vi "Main.vi"() -> ()   [LabVIEW 2019]
uses:
  <vilib>/Platform/TimedLoop/XDataNode/timing_clust.ctl
  <vilib>/Platform/TimedLoop/XDataNode/nitl_modes.ctl
  <vilib>/Platform/TimedLoop/XDataNode/wakeup.ctl
  <vilib>/myRIO/Instrument Drivers/Onboard IO/PWM/typedefs/PWM Reference.ctl
  <vilib>/myRIO/Common/Instrument Driver Framework/Utilities/typedefs/myRIO Generic Hardware Reference.ctl
  <vilib>/myRIO/Common/Instrument Driver Framework/Utilities/typedefs/Hardware Version Enum.ctl
  <vilib>/myRIO/Common/Instrument Driver Framework/Utilities/typedefs/myRIO v1.0 Reference.ctl
  <vilib>/myRIO/Common/Instrument Driver Framework/Utilities/typedefs/Generic FPGA Reference.ctl
  <vilib>/myRIO/Common/Instrument Driver Framework/myRIO v1.0/PWM/typedefs/PWM Channels Enum.ctl
  <vilib>/myRIO/Instrument Drivers/Onboard IO/PWM/typedefs/PWM Configuration.ctl
  <vilib>/userDefined/High Color/nirio_resource_hc.ctl
  <vilib>/myRIO/Instrument Drivers/Onboard IO/DIO/typedefs/DIO Reference.ctl
  <vilib>/myRIO/Common/Instrument Driver Framework/myRIO v1.0/DIO/typedefs/DIO Channels List.ctl
  <vilib>/myRIO/Common/Instrument Driver Framework/myRIO v1.0/DIO/typedefs/DIO Channels Enum.ctl
  <vilib>/myRIO/Common/Instrument Driver Framework/Utilities/vis/Is FPGA Ref Available.vi
  <vilib>/myRIO/Common/Instrument Driver Framework/myRIO v1.0/PWM/vis/myRIO v1.1 Open PWM.vi
  <vilib>/myRIO/Instrument Drivers/Onboard IO/PWM/vis/Set Duty Cycle and Frequency.vi
  <vilib>/myRIO/Common/Instrument Driver Framework/myRIO v1.0/DIO/vis/myRIO v1.1 Open DIO.vi
  <extravilib>/ChannelInstances/Tag-bool/Write With Abort.vi
  <extravilib>/ChannelInstances/Tag-bool/Read With Abort.vi
  <vilib>/myRIO/Common/Instrument Driver Framework/Utilities/vis/Validate Channels.vi
  <vilib>/myRIO/Common/Instrument Driver Framework/myRIO v1.0/PWM/vis/myRIO v1.0 Reserve PWM.vi
  <vilib>/myRIO/Common/Instrument Driver Framework/myRIO v1.0/DIO/vis/myRIO v1.0 Reserve DIO.vi
  <vilib>/myRIO/Common/Instrument Driver Framework/myRIO v1.0/I2C/vis/myRIO v1.0 Close I2C.vi
  <vilib>/myRIO/Common/Instrument Driver Framework/myRIO v1.0/UART/vis/myRIO v1.0 Close UART.vi
  <vilib>/myRIO/Common/Instrument Driver Framework/myRIO v1.0/PWM/vis/myRIO v1.0 Build MUX Configuration PWM.vi
  <vilib>/myRIO/Common/Instrument Driver Framework/myRIO v1.0/Resource Manager/vis/myRIO v1.0 Reserve Channel List.vi
  <vilib>/myRIO/Common/Instrument Driver Framework/myRIO v1.0/DIO/vis/myRIO v1.0 Build MUX Configuration DIO.vi
  <vilib>/myRIO/Common/Instrument Driver Framework/myRIO v1.0/I2C/vis/myRIO v1.0 Unreserve I2C.vi
  <vilib>/myRIO/Common/Instrument Driver Framework/myRIO v1.0/Resource Manager/vis/myRIO v1.0 Create Configuration List.vi
  <vilib>/myRIO/Common/Instrument Driver Framework/myRIO v1.0/Resource Manager/vis/myRIO v1.0 Reserve Channel.vi
  <vilib>/myRIO/Common/Instrument Driver Framework/myRIO v1.0/Resource Manager/vis/myRIO v1.0 Unreserve Channel.vi
  <vilib>/myRIO/Common/Instrument Driver Framework/myRIO v1.0/I2C/vis/myRIO v1.0 Build MUX Configuration I2C.vi
  <vilib>/myRIO/Common/Instrument Driver Framework/myRIO v1.0/Resource Manager/vis/myRIO v1.0 Unreserve Channel List.vi
  <vilib>/myRIO/Common/Instrument Driver Framework/myRIO v1.0/Resource Manager/vis/myRIO v1.0 Build Mutex Name.vi
  <extravilib>/ChannelInstances/Tag-bool/Instantiate.vi
  <extravilib>/ChannelInstances/Tag-bool/EndpointRead.vi
  <vilib>/Utility/VariantDataType/GetNumericInfo.vi
  <vilib>/Utility/error.llb/Error Cluster From Error Code.vi
  <vilib>/myRIO/Common/Instrument Driver Framework/myRIO v1.0/myRIO v1.1 Open.vi
  <vilib>/myRIO/Common/Instrument Driver Framework/Utilities/vis/IO Manager.vi
  <vilib>/myRIO/Common/Instrument Driver Framework/Utilities/vis/Configuration Manager.vi
  <vilib>/myRIO/Common/Instrument Driver Framework/myRIO v1.0/Resource Manager/vis/myRIO v1.0 Configure IO.vi
  <vilib>/myRIO/Common/Instrument Driver Framework/myRIO v1.0/myRIO v1.0 Close.vi
  <vilib>/myRIO/Common/Instrument Driver Framework/myRIO v1.0/PWM/vis/myRIO v1.0 Write PWM.vi
  <vilib>/myRIO/Common/Instrument Driver Framework/myRIO v1.0/DIO/vis/myRIO v1.0 Write DIO.vi
  <vilib>/myRIO/Common/Instrument Driver Framework/myRIO v1.0/I2C/vis/myRIO v1.0 Shutdown I2C.vi
  <vilib>/rvi/errors/niLvFpgaAdjustHostInterfaceError.vi
  <vilib>/FPGAPlugInAG/Dynamic/niLvFpga_Abort_Dynamic.vi
  <vilib>/myRIO/Common/Instrument Driver Framework/Utilities/vis/FPGA Ref Manager.vi
  <vilib>/myRIO/Common/Instrument Driver Framework/myRIO v1.0/myRIO v1.0 Reset FPGA.vi
  <vilib>/myRIO/Common/Instrument Driver Framework/myRIO v1.0/IRQ/vis/myRIO v1.0 IRQ Info FGV.vi
  <vilib>/myRIO/Common/Instrument Driver Framework/myRIO v1.0/IRQ/vis/myRIO v1.0 Timer IRQ Info FGV.vi
  <vilib>/myRIO/Common/Instrument Driver Framework/myRIO v1.0/IRQ/vis/myRIO v1.0 ISR Agent.vi
  <vilib>/myRIO/Instrument Drivers/Utilities/vis/Reset Index.vi
  <vilib>/myRIO/Common/Instrument Driver Framework/myRIO v1.0/Resource Manager/vis/myRIO v1.0 Block Write Resource Manager.vi
  <vilib>/FPGAPlugInAG/Dynamic/niLvFpga_Close_Dynamic.vi
  <extravilib>/ChannelInstances/Tag-bool/Endpoint.vi
  <vilib>/platform/TimedLoop/XDataNode/XDataNode.xnode
  <vilib>/myRIO/Express VI/Onboard IO/PWM/PWM Express VI.xnode
  <vilib>/myRIO/Instrument Drivers/Onboard IO/PWM/vis/myRIO PWM Open.xnode
  <vilib>/myRIO/Express VI/Onboard IO/DO/DO Express VI.xnode
  <vilib>/myRIO/Instrument Drivers/Onboard IO/DIO/vis/myRIO DIO Open.xnode
  <vilib>/rvi/interface/nirviReadWriteControl/nirviReadWriteControl.xnode
  <vilib>/rvi/interface/nirviMethod/nirviMethod.xnode
  <vilib>/rvi/interface/nirviCloseFPGA/nirviCloseFPGA.xnode
  <vilib>/rvi/interface/Simulation/niFpgaSimulationCallBeginRW.vi
  <vilib>/Platform/TimedLoop/XDataNode/XDNodeRunTimeDep.lvlib
  <vilib>/myRIO/Instrument Drivers/Utilities/Utilities.lvlib
  NiFpgaLv.dll
  <extravilib>/ChannelInstances/Tag-bool.lvlib
  <vilib>/myRIO/Instrument Drivers/Onboard IO/PWM/PWM.lvlib
  <vilib>/myRIO/Instrument Drivers/Onboard IO/DIO/DIO.lvlib
  <vilib>/myRIO/Instrument Drivers/Onboard IO/I2C/I2C.lvlib
panel:
  out "Encoder Position (Degrees) 2":dbl
  out "Duty Cycle PWM":dbl(graph)
  in  "Inner PID T/F":bool
  in  "D_i":dbl
  in  "I_i":dbl
  in  "P_i":dbl
  in  "Log file path":path
  out "Duty Cycle":dbl
  in  "Angle limit (degrees)":i32
  in  "D_o":dbl
  in  "I_o":dbl
  in  "P_o":dbl
  in  "Speed (km/h)":dbl
  out "Combined loop duration time (us)":i64
  in  "Loop durations":T1(tab)
  out "IMU Data gathering duration(us)":i64(graph)
  out "Encoder data gathering duration(us)":i64(graph)
  out "Steering Motor duration(us)":i64(graph)
  out "E-Stop loop duration (us)":i64(graph)
  in  "GO":bool
  in  "E-stop":bool
  out "Indicator":bool
  in  "Encoder Position Reset":bool
  out "Encoder Velocity (deg/s)":dbl
  out "Encoder Acceleration (deg/s^2)":dbl
  out "Encoder Position (Degrees)":dbl
  out "IMU Gyro Chart":cluster{dbl, dbl, dbl}(graph)
  out "IMU Acc Chart":cluster{dbl, dbl, dbl}(graph)
  # "Steering Motor"
  # "Forward Motor"
  # "Outer"
  # "(2)"
  # "Inner"
  # "Start Motors"
  # "(3)"
  # "(1)"
  # "(4)"
  # "(6)"
  # "(7)"
  # "(5)"
  # "(8)"
  # "(8)"
  # "(8)"
  # "(8)"
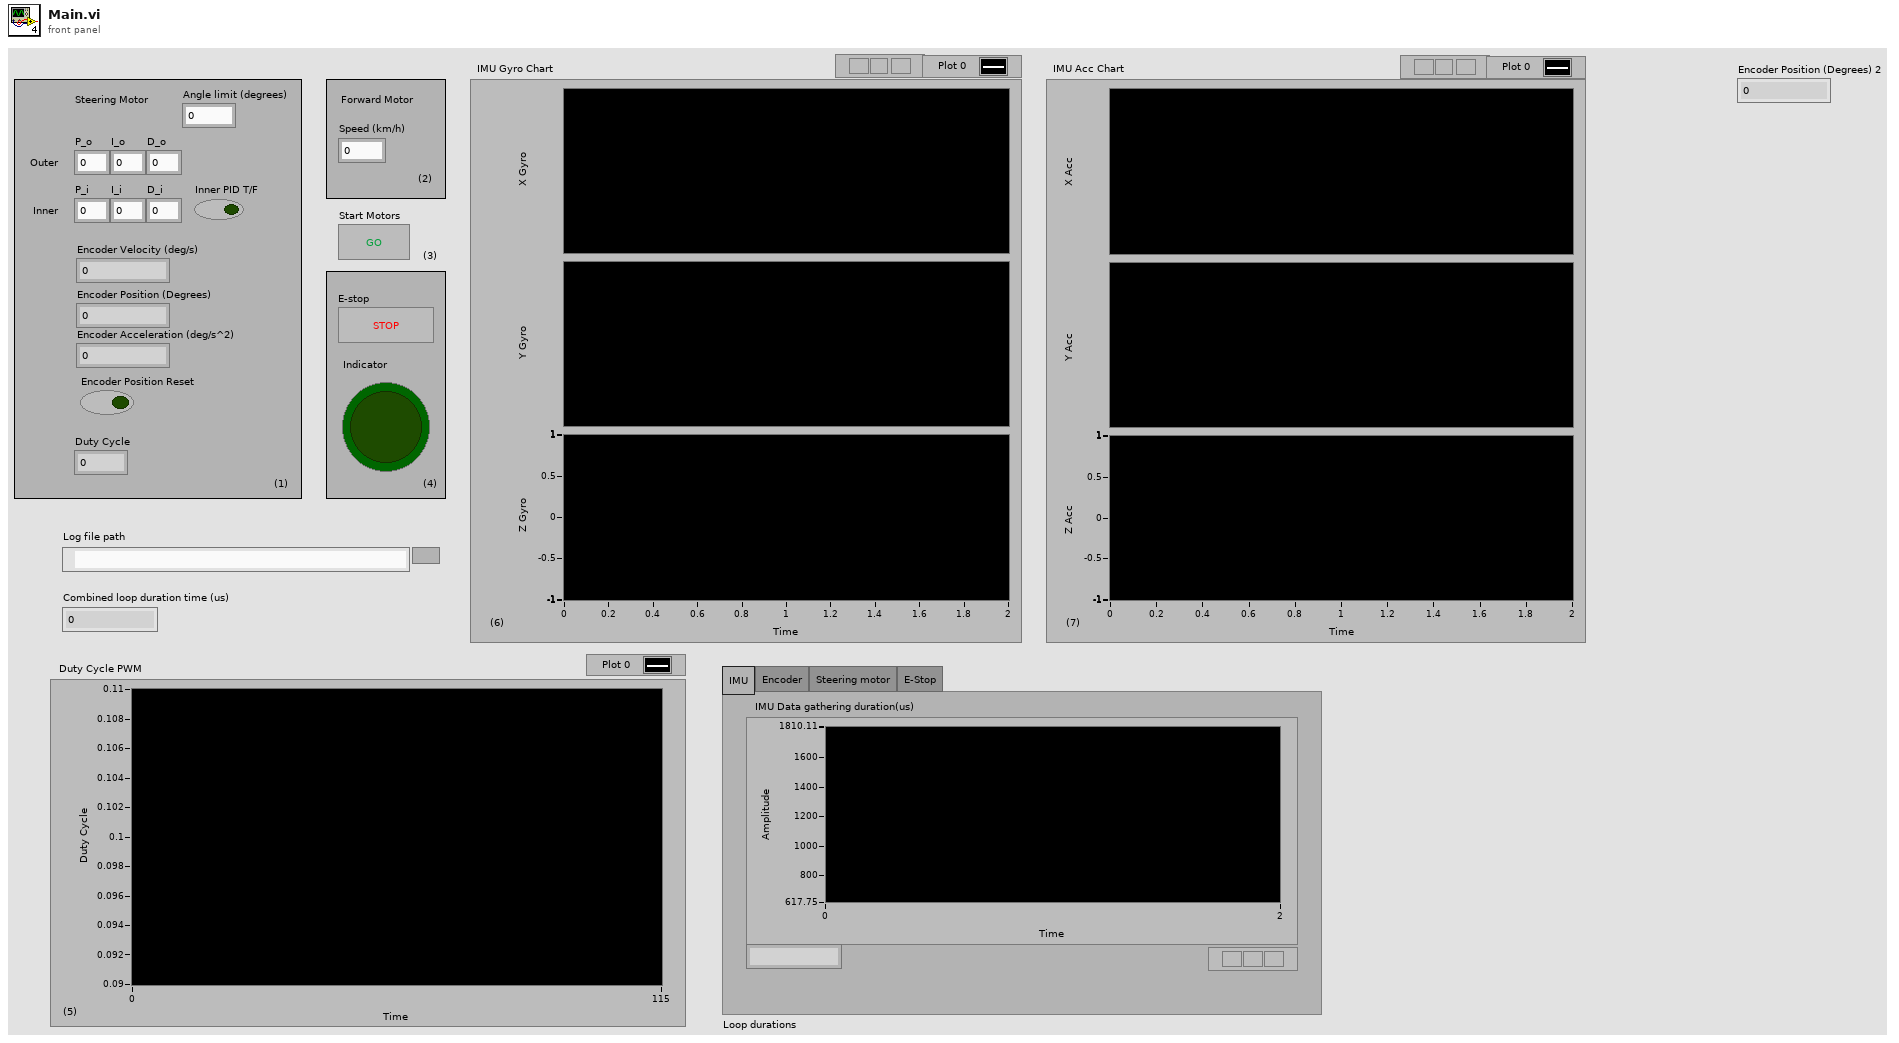
[diagram p1: front panel]
types:
  T1 = enum32{"IMU", "Encoder", "Steering motor", "E-Stop"}
  T2 = enum16{"open", "open or create", "create or replace", "create", "open (read-only)"}
  T3 = typedef "XDNodeRunTimeDep.lvlib/timing_clust.ctl" = cluster{"Expected End [f-1]":u64, "Actual End [f-1]":u64, "Finished Late? [f-1]":bool, "Expected End [i-1]":u64, "Actual End [i-1]":u64, "Finished Late? [i-1]":bool, "Expected Start [i]":u64, "Actual Start [i]":u64, "Expected Start [f]":u64, "Actual Start [f]":u64, "Source Name":string, "Structure Name":string, "Period":i64, "Deadline":i64, "Offset":i64, "Start":i64, "Priority":i32, "Timeout":i32, "Mode":T4, "Wakeup Reason":T5, "Error":errorcluster, "Source Type":string, "Secondary Source Type":string, "Global End Time":u64, "Global Start Time":u64, "Frame Duration":u64, "Iteration Duration":u64, "Assigned CPU":i32, "I/O Scan Engine Mode":u32}
  T4 = typedef "XDNodeRunTimeDep.lvlib/nitl_modes.ctl" = enum32{"No Change", "Process missed periods, maintain original phase", "Discard missed periods, maintain original phase", "Process missed periods, ignore original phase", "Discard missed periods, ignore original phase"}
  T5 = typedef "XDNodeRunTimeDep.lvlib/wakeup.ctl" = enum32{"Normal", "Aborted", "Asynchronous wakeup", "Timing source error", "Timed loop error", "Timeout"}
  T6 = typedef "I2C.lvlib/I2C Reference.ctl" = cluster{"myRIO Reference":T7, "I2C Channels Enum":T11, "I2C Configuration":T12}
  T7 = typedef "myRIO Generic Hardware Reference.ctl" = cluster{"myRIO Model":T8, "myRIO Hardware Reference":T9}
  T8 = typedef "Hardware Version Enum.ctl" = enum16{"Unknown", "myRIO-1900", "myRIO-1950", "roboRIO", "NI ELVIS RIO CM", "ELVIS III"}
  T9 = typedef "myRIO v1.0 Reference.ctl" = cluster{"Generic FPGA Reference":T10, "Allow multiple opens":bool}
  T10 = typedef "Generic FPGA Reference.ctl" = refnum<k20>
  T11 = typedef "I2C Channels Enum.ctl" = enum16{"Not Connected", "A/I2C", "B/I2C", "I2C/I2C"}
  T12 = typedef "I2C.lvlib/I2C Configuration.ctl" = cluster{"I2C Transfer Rate":T13}
  T13 = typedef "I2C.lvlib/I2C Transfer Rate.ctl" = enum16{"Standard mode (100 kbps)", "Fast mode (400 kbps)"}
  T14 = typedef "Tag-bool.lvlib/))Channel.ctl" = refnum<queue>
  T15 = typedef "PWM.lvlib/PWM Reference.ctl" = cluster{"myRIO Reference":T7, "PWM Channels Enum":T16, "PWM Configuration":T17}
  T16 = typedef "PWM Channels Enum.ctl" = enum16{"Not Connected", "C/PWM0", "C/PWM1", "A/PWM0", "A/PWM1", "A/PWM2", "A/PWM3", "A/PWM4", "A/PWM5", "A/PWM6", "A/PWM7", "A/PWM8", "A/PWM9", "A/PWM10", "A/PWM11", "A/PWM12", "A/PWM13", "A/PWM14", "A/PWM15", "A/PWM16", "A/PWM17", "A/PWM18", "A/PWM19", "B/PWM0", "B/PWM1", "B/PWM2", "B/PWM3", "B/PWM4", "B/PWM5", "B/PWM6", "B/PWM7", "B/PWM8", "B/PWM9", "B/PWM10", "B/PWM11", "B/PWM12", "B/PWM13", "B/PWM14", "B/PWM15", "B/PWM16", "B/PWM17", "B/PWM18", "B/PWM19", "PWM/PWM0", "PWM/PWM1", "PWM/PWM2", "PWM/PWM3", "PWM/PWM4", "PWM/PWM5", "PWM/PWM6", "PWM/PWM7", "PWM/PWM8", "PWM/PWM9"}
  T17 = typedef "PWM.lvlib/PWM Configuration.ctl" = cluster{"Frequency":dbl, "Duty Cycle":dbl}
  T18 = typedef "nirio_resource_hc.ctl" = tag
  T19 = typedef "DIO.lvlib/DIO Reference.ctl" = cluster{"myRIO Reference":T7, "DIO Channels List":T20}
  T20 = typedef "DIO Channels List.ctl" = T21[]
  T21 = typedef "DIO Channels Enum.ctl" = enum16{"Not Connected", "C/DIO0", "C/DIO1", "C/DIO2", "C/DIO3", "C/DIO4", "C/DIO5", "C/DIO6", "C/DIO7", "A/DIO0", "A/DIO1", "A/DIO2", "A/DIO3", "A/DIO4", "A/DIO5", "A/DIO6", "A/DIO7", "A/DIO8", "A/DIO9", "A/DIO10", "A/DIO11", "A/DIO12", "A/DIO13", "A/DIO14", "A/DIO15", "A/DIO16", "A/DIO17", "A/DIO18", "A/DIO19", "B/DIO0", "B/DIO1", "B/DIO2", "B/DIO3", "B/DIO4", "B/DIO5", "B/DIO6", "B/DIO7", "B/DIO8", "B/DIO9", "B/DIO10", "B/DIO11", "B/DIO12", "B/DIO13", "B/DIO14", "B/DIO15", "B/DIO16", "B/DIO17", "B/DIO18", "B/DIO19", "LED0", "LED1", "LED2", "LED3", "Button0", "DIO/DIO0", "DIO/DIO1", "DIO/DIO2", "DIO/DIO3", "DIO/DIO4", "DIO/DIO5", "DIO/DIO6", "DIO/DIO7", "DIO/DIO8", "DIO/DIO9", "SPI/CS0", "SPI/CS1", "SPI/CS2", "SPI/CS3", "LED RADIO (Green)", "LED RADIO (Red)", "LED COMM (Green)", "LED COMM (Red)", "LED MODE (Green)", "LED MODE (Red)"}
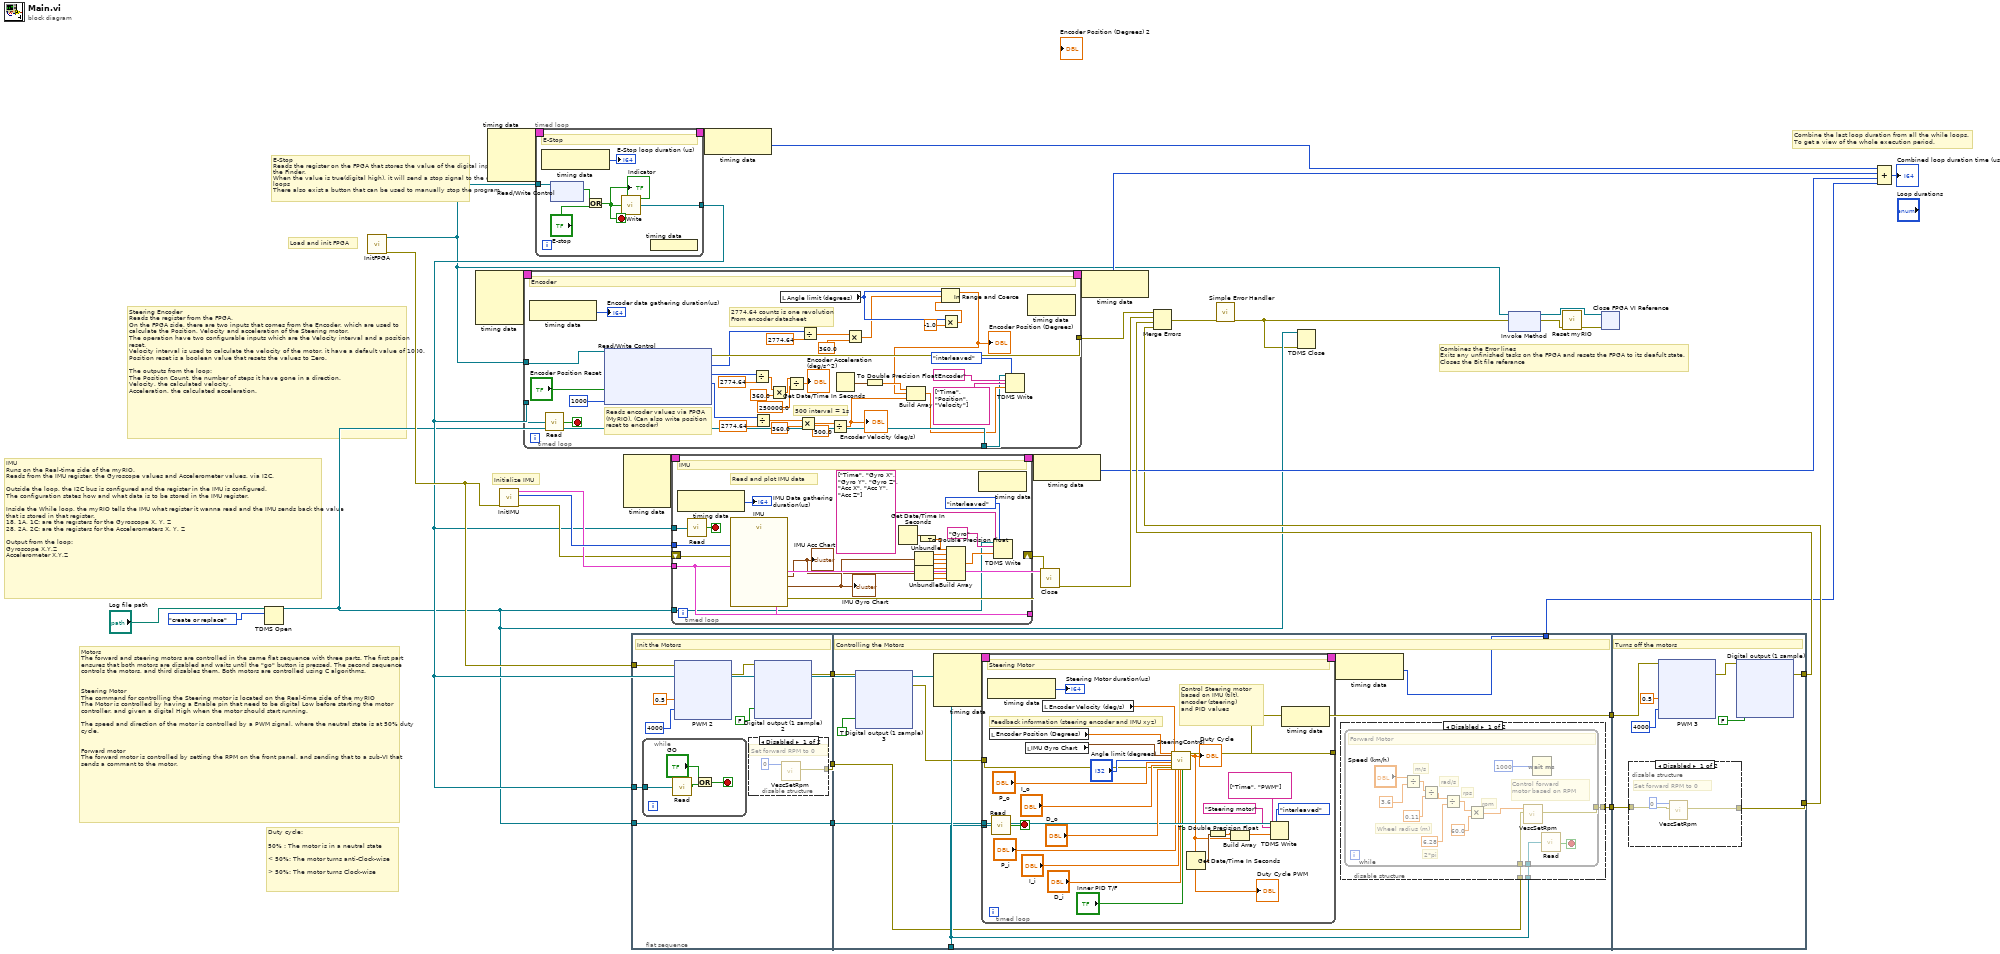
[diagram p0: block diagram]
diagram:
  # "Duty cycle:\n\n50% : The motor is in a neutral state\n\n< 50%: The motor turns anti-Clock-wise\n\n> 50%: The motor turns Clock-wise"
  # "Initialize IMU"
  # "Load and init FPGA"
  # "Combines the Error lines\nExits any unfinished tasks on the FPGA and resets the FPGA to its deafult state.\nCloses the Bit file referance"
  # "Combine the last loop duration from all the while loops.\nTo get a view of the whole execution period."
  # "Motors\nThe forward and steering motors are controlled in the same flat sequence with three parts. The first part ensures that both motors are disabled and waits until the \"go\" button is pressed. The second sequence controls the motors, and third disables them. Both motors are controlled using C algorithms.\n\n\nSteering Motor\nThe command for controlling the Steering motor is located on the Real-time side of the myRIO\nThe Motor is controlled by having a Enable pin that need to be digital Low before starting the motor controller, and given a digital High when the motor should start running.\n\nThe speed and direction of the motor is controlled by a PWM signal, where the neutral state is at 50% duty cycle.\n\n\nForward motor\nThe forward motor is controlled by setting the RPM on the front panel, and sending that to a sub-VI that sends a commant to the motor."
  # "IMU\nRuns on the Real-time side of the myRIO.\nReads from the IMU register, the Gyroscope values and Accelerometer values, via I2C.\n\nOutside the loop, the I2C bus is configured and the register in the IMU is configured.\nThe configuration states how and what data is to be stored in the IMU register.\n\nInside the While loop, the myRIO tells the IMU what register it wanna read and the IMU sends back the value that is stored in that register.\n18, 1A, 1C: are the registers for the Gyroscope X, Y, Z\n28, 2A, 2C: are the registers for the Accelerometers X, Y, Z\n\nOutput from the loop:\nGyroscope X,Y,Z\nAccelerometer X,Y,Z"
  # "Steering Encoder\nReads the register from the FPGA. \nOn the FPGA side, there are two inputs that comes from the Encoder, which are used to calculate the Position, Velocity and acceleration of the Steering motor.\nThe operation have two configurable inputs which are the Velocity interval and a position reset.\nVelocity interval is used to calculate the velocity of the motor, it have a default value of 1000.\nPosition reset is a boolean value that resets the values to Zero.\n\nThe outputs from the loop:\nThe Position Count, the number of steps it have gone in a direction. \nVelocity, the calculated velocity.\nAcceleration, the calculated acceleration."
  # "E-Stop\nReads the register on the FPGA that stores the value of the digital input from the Finder.\nWhen the value is true(digital high), it will send a stop signal to the other while loops\nThere also exist a button that can be used to manually stop the program."
  n1 = TDMS Open(10:T2."create or replace" ("operation (0:open)"), 11:"Log file path") -> (3:w5:refnum<k34>)  [unwired: 5 in, 1 out]
  n2 = call "InitFPGA.vi"() -> ("error out"=w20:errorcluster, "Refnum out"=w1:refnum<k20>)  [unwired: 10 in]
  n3 = node-c288() -> (w33:T3)  [unwired: 4 in]
  n4 = node-c288() -> (w27:T3)  [unwired: 4 in]
  n5 = call "InitIMU.vi"("error in (no error)"=w20) -> ("error out"=w15:errorcluster, "Acc/Gyro  address"=w22:u8, "I2C Ref Out"=w21:T6)  [unwired: 8 in]
  n6 = timed-loop {
    timing: w27 -> [_]
    timing-out: [_] -> w26
    tunnel: w1 -> [w42]
    tunnel: [w41] -> w13
    stop <- w37 stop-if-true
    # "E-Stop"
    n7 = node-c288() -> (→"E-Stop loop duration (us)":i64)  [unwired: 1 in]
    n8 = xnode "Read/Write Control"("FPGA VI Reference In"=w42) -> ("E-Stop"=w40:bool)  [unwired: 1 in, 2 out]
    n9 = Or(x=w40, y="E-stop") -> (x .or. y?=w37:bool)
    "Indicator" <- w37
    n10 = call <vilib>:"Write.vi"("element"=w37) -> ("channel"=w41:T14)  [unwired: 1 out]
    n11 = node-c288() -> ()  [unwired: 1 out]
  }
  n12 = timed-loop {
    timing: w33 -> [_]
    timing-out: [_] -> w32
    tunnel: w1 -> [w82]
    tunnel: [w81] -> w31
    tunnel: w13 -> [w77]
    tunnel: w5 -> [w72]
    stop <- w76 stop-if-true
    # "500 interval = 1s"
    # "2774,64 counts is one revolution\nFrom encoder datasheet"
    # "Reads encoder values via FPGA\n(MyRIO). (Can also write position\nreset to encoder)"
    # "Encoder"
    n13 = node-c288() -> (→"Encoder data gathering duration(us)":i64)  [unwired: 1 in]
    n14 = call <extravilib>:"Read.vi"("channel"=w77) -> ("element"=w76:bool)  [unwired: 1 in, 1 out]
    n15 = xnode "Read/Write Control"("FPGA VI Reference In"=w82, "Position Reset"="Encoder Position Reset", "Velocity Interval (uSec)"=u32 1000) -> ("error out"=w81:errorcluster, "Position (Counts)"=w68:i32, "Acceleration (Counts/Interval)"=w56:i32, "Velocity (Counts/Interval)"=w61:i32)  [unwired: 1 in, 1 out]
    n16 = Divide(x=w56, y=2774.64) -> (x/y=w54:dbl)
    n17 = Divide(x=w61, y=2774.64) -> (x/y=w62:dbl)
    n18 = Multiply(x=w54, y=360.0) -> (x*y=w53:dbl)
    n19 = local read "Angle limit (degrees)"() -> (w49:i32)
    n20 = Divide(x=w53, y=250000.0) -> (x/y=→"Encoder Acceleration (deg/s^2)":dbl)
    n21 = Multiply(x=w62, y=360.0) -> (x*y=w60:dbl)
    n22 = Divide(x=w68, y=2774.64) -> (x/y=w65:dbl)
    n23 = Divide(x=w60, y=500.0) -> (x/y=w58:dbl)
    "Encoder Velocity (deg/s)" <- w58
    n24 = Get Date/Time In Seconds() -> (seconds since 1Jan1904=w70:timestamp)
    n25 = Multiply(x=w65, y=360.0) -> (x*y=w47:dbl)
    n26 = To Double Precision Float(number=w70) -> (double precision float=w71:dbl)
    n27 = Multiply(x=w49, y=-1.0) -> (x*y=w50:dbl)
    n28 = In Range and Coerce(upper limit=w49, x=w47, lower limit=w50) -> (coerced(x)=w46:dbl)  [unwired: 1 out]
    "Encoder Position (Degrees)" <- w46
    n29 = Build Array(w71, w46, w58) -> (w73:dbl[])
    n30 = TDMS Write(0:w72, 1:enum16{"decimated", "interleaved"}."interleaved" ("data layout (0:decimated)"), 5:"Encoder" ("group name in (Untitled)"), 7:string[] ["Time", "Position", "Velocity"] ("channel name(s) in (Untitled)"), 9:w73) -> ()  [unwired: 1 in, 4 out]
    n31 = node-c288() -> ()  [unwired: 1 in, 1 out]
  }
  n32 = node-c288() -> (w29:T3)  [unwired: 4 in]
  n33 = flat-sequence {
    tunnel: [w93] -> w25
    tunnel: w20 -> [w91]
    tunnel: w13 -> [w89]
    tunnel: [w87] -> w12
    tunnel: w5 -> [w88]
    tunnel: [w88] -> w6
    tunnel: w25 -> [w181]
    tunnel: [w178] -> w3
    tunnel: w13 -> [w175]
    tunnel: w12 -> [w171]
    tunnel: [w174] -> w11
    tunnel: [w173] -> w9
    tunnel: w6 -> [w172]
    tunnel: [w270] -> w17
    tunnel: w11 -> [w266]
    tunnel: [w264] -> w10
    tunnel: w9 -> [w265]
    frame #0 {
      # "Init the Motors"
      n34 = while {
        tunnel: w89 -> [w97]
        stop <- w100 stop-if-true
        n35 = call <extravilib>:"Read.vi"("channel"=w97) -> ("element"=w98:bool)  [unwired: 1 in, 1 out]
        n36 = Or(x="GO", y=w98) -> (x .or. y?=w100:bool)
      }
      n37 = xnode "PWM 2"("Duty Cycle"=0.5, "Frequency [Hz]"=4000, "error in (no error)"=w91) -> ("error out"=w94:errorcluster)
      n38 = disable-structure shown="Disabled" {
        disable-tunnel: [w95 _] -> w87
        frame Disabled {
          # "Set forward RPM to 0"
          n39 = call "VescSetRpm.vi"("Speed (rpm)"=0) -> ("error out"=w95:errorcluster)  [unwired: 10 in]
        }
        frame Enabled {
        }
      }
      n40 = xnode "Digital output (1 sample) 2"("B/DIO4 (Pin 19)"=FALSE ("B/DIO1 (Pin 13)"), "error in (no error)"=w94) -> ("error out"=w93:errorcluster)
    }
    frame #1 {
      # "Controlling the Motors"
      n41 = xnode "Digital output (1 sample) 3"("B/DIO4 (Pin 19)"=TRUE ("B/DIO1 (Pin 13)"), "error in (no error)"=w181) -> ("error out"=w177:errorcluster)
      n42 = node-c288() -> (w180:T3)  [unwired: 4 in]
      n43 = timed-loop {
        tunnel: w177 -> [w199]
        timing: w180 -> [_]
        timing-out: [_] -> w179
        tunnel: w175 -> [w215]
        tunnel: [w213] -> w173
        tunnel: w172 -> [w212]
        stop <- w222 stop-if-true
        # "Feedback information (steering encoder and IMU xyz)"
        # "Control Steering motor\nbased on IMU (tilt), \nencoder (steering)\nand PID values"
        # "Steering Motor"
        n44 = node-c288() -> (→"Steering Motor duration(us)":i64)  [unwired: 1 in]
        n45 = local read "Encoder Position (Degrees)"() -> (w219:dbl)
        n46 = call <extravilib>:"Read.vi"("channel"=w215) -> ("element"=w222:bool)  [unwired: 1 in, 1 out]
        n47 = local read "IMU Gyro Chart"() -> (w220:cluster{dbl, dbl, dbl})
        n48 = local read "Encoder Velocity (deg/s)"() -> (w201:dbl)
        n49 = call "SteeringControl.vi"("Position (Degrees)"=w219, "Cluster"=w220, "Limit (degrees)"="Angle limit (degrees)", "P_o gain"="P_o", "I_o gain"="I_o", "error in (no error)"=w199, "D_o gain"="D_o", "Velocity (deg/s)"=w201, "P_i gain"="P_i", "I_i gain"="I_i", "D_i gain"="D_i", "Inner PID T/F"="Inner PID T/F") -> ("error out"=w213:errorcluster, "PWM Out"=w200:dbl)  [unwired: 14 in]
        "Duty Cycle" <- w200
        "Duty Cycle PWM" <- w200
        n50 = Get Date/Time In Seconds() -> (seconds since 1Jan1904=w208:timestamp)
        n51 = To Double Precision Float(number=w208) -> (double precision float=w209:dbl)
        n52 = Build Array(w209, w200) -> (w210:dbl[])
        n53 = TDMS Write(0:w212, 1:enum16{"decimated", "interleaved"}."interleaved" ("data layout (0:decimated)"), 5:"Steering motor" ("group name in (Untitled)"), 7:string[] ["Time", "PWM"] ("channel name(s) in (Untitled)"), 9:w210) -> ()  [unwired: 1 in, 4 out]
        n54 = node-c288() -> ()  [unwired: 1 in, 1 out]
      }
      n55 = node-c288(w179) -> (w178:i64)
      n56 = disable-structure shown="Disabled" {
        disable-tunnel: w175 -> [w184 _]
        disable-tunnel: [w183 _] -> w174
        disable-tunnel: w171 -> [w182 _]
        frame Disabled {
          n57 = while "Timed Loop" {
            tunnel: w184 -> [w197]
            tunnel: w182 -> [w186]
            tunnel: [w185] -> w183
            stop <- w198 stop-if-true
            # "2*pi"
            # "rpm"
            # "rps"
            # "rad/s"
            # "Wheel radius (m)"
            # "m/s"
            # "Control forward\nmotor based on RPM"
            # "Forward Motor"
            n58 = Divide(x="Speed (km/h)", y=3.6) -> (x/y=w193:dbl)
            n59 = Divide(x=w193, y=0.11) -> (x/y=w191:dbl)
            n60 = Divide(x=w191, y=6.28) -> (x/y=w190:dbl)
            n61 = Multiply(x=w190, y=60.0) -> (x*y=w188:dbl)
            n62 = call "VescSetRpm.vi"("error in (no error)"=w186, "Speed (rpm)"=w188) -> ("error out"=w185:errorcluster)  [unwired: 9 in]
            n63 = Wait (ms)(milliseconds to wait=1000) -> ()  [unwired: 1 out]
            n64 = call <extravilib>:"Read.vi"("channel"=w197) -> ("element"=w198:bool)  [unwired: 1 in, 1 out]
          }
        }
        frame Enabled {
        }
      }
    }
    frame #2 {
      # "Turns off the motors"
      n65 = disable-structure shown="Disabled" {
        disable-tunnel: w266 -> [w273 _]
        disable-tunnel: [w272 _] -> w264
        frame Disabled {
          # "Set forward RPM to 0"
          n66 = call "VescSetRpm.vi"("error in (no error)"=w273, "Speed (rpm)"=0) -> ("error out"=w272:errorcluster)  [unwired: 9 in]
        }
        frame Enabled {
        }
      }
      n67 = xnode "PWM 3"("Duty Cycle"=0.5, "Frequency [Hz]"=4000, "error in (no error)"=w265) -> ("error out"=w268:errorcluster)
      n68 = xnode "Digital output (1 sample)"("B/DIO4 (Pin 19)"=FALSE ("B/DIO1 (Pin 13)"), "error in (no error)"=w268) -> ("error out"=w270:errorcluster)
    }
  }
  n69 = timed-loop {
    timing: w29 -> [_]
    timing-out: [_] -> w28
    tunnel: w22 -> [w366]
    tunnel: w21 -> [w363]
    shift-right: [w360] -> w16
    shift-left: w15 -> [w365]
    tunnel: [w363] -> w19
    tunnel: w13 -> [w362]
    tunnel: w5 -> [w355]
    stop <- w361 stop-if-true
    # "Read and plot IMU data"
    # "IMU"
    n70 = node-c288() -> (→"IMU Data gathering duration(us)":i64)  [unwired: 1 in]
    n71 = call <extravilib>:"Read.vi"("channel"=w362) -> ("element"=w361:bool)  [unwired: 1 in, 1 out]
    n72 = call "IMU.vi"("error in (no error)"=w365, "Acc/Gyro  address"=w366, "I2C Ref"=w363) -> ("error out"=w360:errorcluster, "IMU Acc"=w348:cluster{dbl, dbl, dbl}, "IMU Gyro"=w359:cluster{dbl, dbl, dbl})  [unwired: 6 in]
    "IMU Acc Chart" <- w348
    "IMU Gyro Chart" <- w359
    n73 = Get Date/Time In Seconds() -> (seconds since 1Jan1904=w353:timestamp)
    n74 = Unbundle(w359) -> (w358:dbl, w350:dbl, w349:dbl)
    n75 = Unbundle(w348) -> (w347:dbl, w346:dbl, w345:dbl)
    n76 = To Double Precision Float(number=w353) -> (double precision float=w354:dbl)
    n77 = Build Array(w354, w358, w350, w349, w347, w346, w345) -> (w356:dbl[])
    n78 = node-c288() -> ()  [unwired: 1 in, 1 out]
    n79 = TDMS Write(0:w355, 1:enum16{"decimated", "interleaved"}."interleaved" ("data layout (0:decimated)"), 5:"Gyro" ("group name in (Untitled)"), 7:string[] ["Time", "Gyro X", "Gyro Y", "Gyro Z", "Acc X", "Acc Y", "Acc Z"] ("channel name(s) in (Untitled)"), 9:w356) -> ()  [unwired: 1 in, 4 out]
  }
  n80 = node-c288(w26) -> (w2:i64)
  n81 = node-c288(w28) -> (w14:i64)
  n82 = call <vilib>:"Close.vi"("error in (no error)"=w16, "I2C Ref In"=w19) -> ("error out"=w18:errorcluster)  [unwired: 9 in]
  n83 = node-c288(w32) -> (w24:i64)
  n84 = Merge Errors(w31, w18, w17, w10) -> (w30:errorcluster)
  n85 = call <vilib>:"Simple Error Handler.vi"("error in (no error)"=w30) -> ("error out"=w4:errorcluster)  [unwired: 4 in, 4 out]
  n86 = TDMS Close(8:w4, 11:w5) -> ()  [unwired: 2 out]
  n87 = xnode "Invoke Method"("FPGA VI Reference In"=w1, "error in"=w4) -> ("FPGA VI Reference Out"=w36:refnum<k20>, "error out"=w34:errorcluster)
  n88 = call <vilib>:"Reset myRIO.vi"("error in (no error)"=w34) -> ("error out"=w35:errorcluster)  [unwired: 10 in]
  n89 = xnode "Close FPGA VI Reference"("FPGA VI Reference In"=w36, "error in"=w35) -> ()  [unwired: 1 out]
  n90 = Compound Arithmetic op=ADD(w2, w24, w14, w3) -> (→"Combined loop duration time (us)":i64)
